vi "Open All Relays.vi"(8 "error in":errorcluster, 11 "2575 in":refnum<class "2575.lvclass">) -> (0 "error out":errorcluster, 3 "2575 out":refnum<class "2575.lvclass">)   [LabVIEW 2019, in "2575.lvlib" / "2575.lvclass"]
uses:
  Library/2575.lvclass
  Library/2575.lvclass/2575.ctl
  builds/Instruments/SwitchMatrix.lvlibp/Library/SwitchMatrix.lvclass
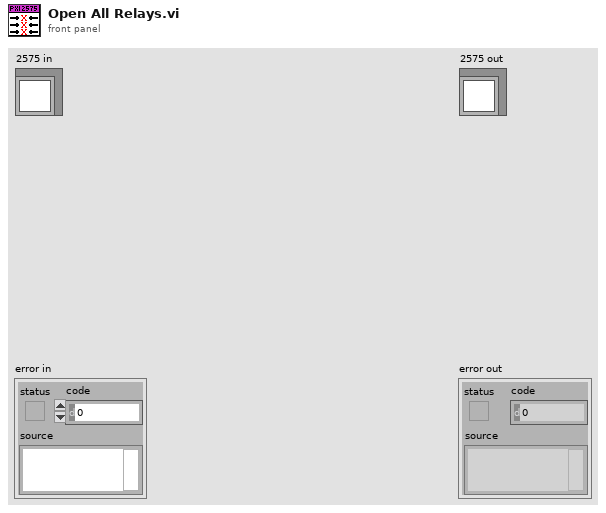
[diagram p1: front panel]
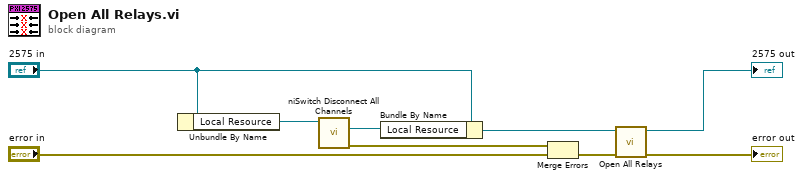
[diagram p0: block diagram]
diagram:
  n1 = Unbundle By Name("2575 in") -> ("Local Resource"=w7:refnum<k15>)
  n2 = call <instrlib>:"niSwitch Disconnect All Channels.vi"("instrument handle"=w7) -> ("error out"=w9:errorcluster, "instrument handle out"=w6:refnum<k15>)  [unwired: 9 in]
  n3 = Bundle By Name(cluster="2575 in", "Local Resource"=w6) -> (w2:refnum<class "2575.lvclass">)
  n4 = Merge Errors(w9, "error in") -> (w4:errorcluster)
  n5 = call-parent "Open All Relays.vi"("error in"=w4, "SwitchMatrix in"=w2) -> ("error out"=→"error out":errorcluster, "SwitchMatrix out"=→"2575 out":refnum<class "2575.lvclass">)  [unwired: 8 in]
